vi "Measure DC Volts4.vi"(10 "measurementservice_DMMConfigRequest_Data":T1) -> (0 "error out":errorcluster, 2 "Measurement Array (Volts)":dbl[](array[numeric]))   [LabVIEW 2019, in "HVC4.lvlib" / "HVC4.lvclass"]
uses:
  HVC4 Class/HVC4.lvclass
  <instrlib>/niDMM/nidmm.llb/niDMM Configure Measurement Digits.vi
  HVC4 Class/RPC Messages/measurementservice_DMMConfigRequest/measurementservice_DMMConfigRequest_Data.ctl
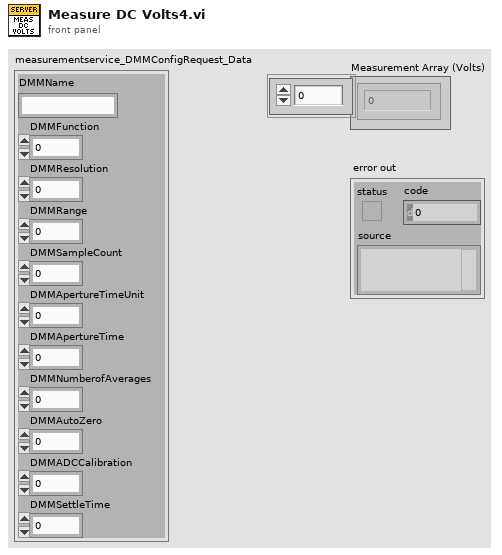
[diagram p1: front panel]
types:
  T1 = typedef "HVC4.lvlib/HVC4.lvclass/measurementservice_DMMConfigRequest_Data.ctl" = cluster{"DMMName":string, "DMMFunction":i32, "DMMResolution":sgl, "DMMRange":sgl, "DMMSampleCount":i32, "DMMApertureTimeUnit":i32, "DMMApertureTime":sgl, "DMMNumberofAverages":i32, "DMMAutoZero":i32, "DMMADCCalibration":i32, "DMMSettleTime":sgl}
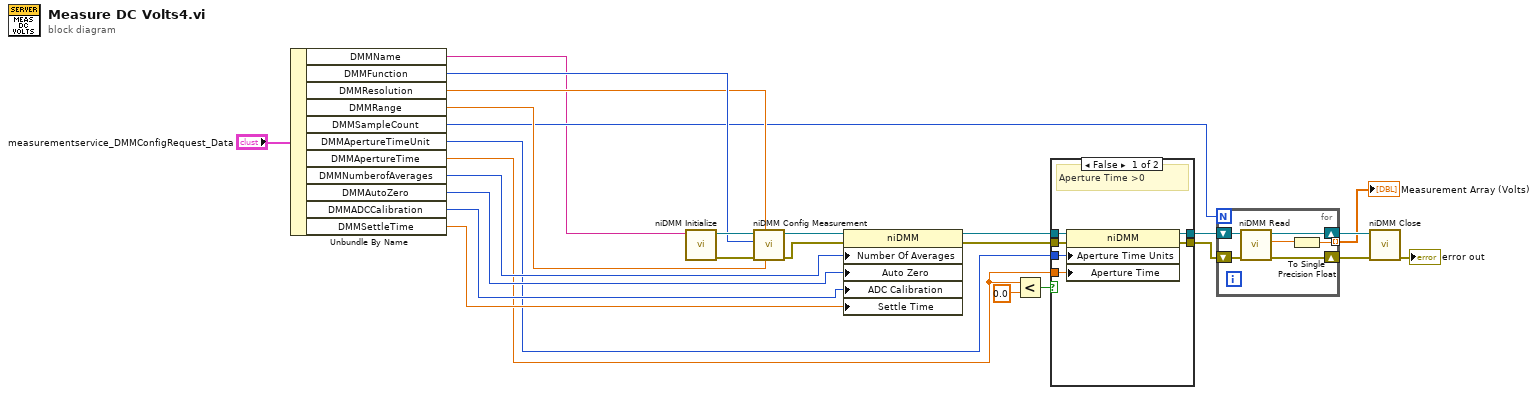
[diagram p0: block diagram]
diagram:
  n1 = Unbundle By Name("measurementservice_DMMConfigRequest_Data") -> ("DMMName"=w1:string, "DMMFunction"=w21:i32, "DMMResolution"=w20:sgl, "DMMRange"=w19:sgl, "DMMSampleCount"=w18:i32, "DMMApertureTimeUnit"=w5:i32, "DMMApertureTime"=w4:sgl, "DMMNumberofAverages"=w15:i32, "DMMAutoZero"=w14:i32, "DMMADCCalibration"=w13:i32, "DMMSettleTime"=w12:sgl)
  n2 = call <instrlib>:"niDMM Initialize.vi"("Instrument Descriptor"=w1) -> ("error out"=w24:errorcluster, "instrument handle out"=w25:refnum<k15>)  [unwired: 9 in]
  n3 = call-poly <instrlib>:"niDMM Config Measurement.vi"("Range"=w19, "Resolution in Digits"=w20, "error in (no error)"=w24, "Function"=w21, "instrument handle"=w25) -> ("error out"=w16:errorcluster, "instrument handle out"=w17:refnum<k15>)  [unwired: 5 in]
  n4 = property class="niDMM"(reference=w17, error in=w16, "Number Of Averages"=w15, "Auto Zero"=w14, "ADC Calibration"=w13, "Settle Time"=w12) -> (reference out=w11:refnum<k15>, error out=w10:errorcluster)
  n5 = Less?(x=w4, y=0.0 ("Configuration:Advanced:Aperture Time")) -> (x < y?=w6:bool)
  n6 = case shown="False" w6 {
    tunnel: w11 -> [w32 w34]
    tunnel: w10 -> [w31 w33]
    tunnel: [w30 w34] -> w9
    tunnel: [w29 w33] -> w8
    tunnel: w5 -> [w28 _]
    tunnel: w4 -> [w27 _]
    frame False {
      # "Aperture Time >0"
      n7 = property class="niDMM"(reference=w32, error in=w31, "Aperture Time Units"=w28, "Aperture Time"=w27) -> (reference out=w30:refnum<k15>, error out=w29:errorcluster)
    }
    frame True {
      # "Aperture Time <0"
    }
  }
  n8 = for {
    N: w18 -> [_]
    tunnel: [w35] -> w3 mode=indexing
    shift-right: [w39] -> w22
    shift-left: w8 -> [w38]
    shift-right: [w40] -> w23
    shift-left: w9 -> [w37]
    n9 = call <instrlib>:"niDMM Read.vi"("error in (no error)"=w38, "instrument handle"=w37) -> ("error out"=w39:errorcluster, "Measurement"=w36:dbl, "instrument handle out"=w40:refnum<k15>)  [unwired: 7 in]
    n10 = To Single Precision Float(number=w36) -> (single precision float=w35:sgl)
  }
  "Measurement Array (Volts)" <- w3
  n11 = call <instrlib>:"niDMM Close.vi"("error in (no error)"=w22, "instrument handle"=w23) -> ("error out"=→"error out":errorcluster)  [unwired: 9 in]
